vi "Get Maximum Button Width Vertical Toolbar.vi"(10 "Button Width":i32, 11 "All Icon Bounds":T1[](array[typedef])) -> (3 "Maximum Button Width":i32)   [LabVIEW 2011]
doc: "-------------\nDeveloped by Brian Hoover (hooovahh)"
uses:
  <vilib>/Utility/miscctls.llb/LVRectTypeDef.ctl
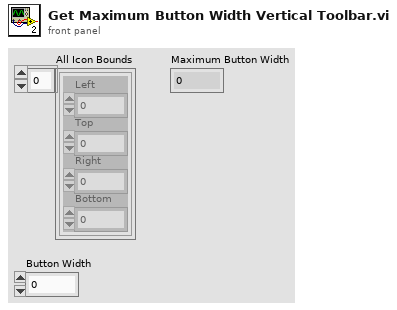
[diagram p1: front panel]
types:
  T1 = typedef "LVRectTypeDef.ctl" = cluster{"Left":i16, "Top":i16, "Right":i16, "Bottom":i16}
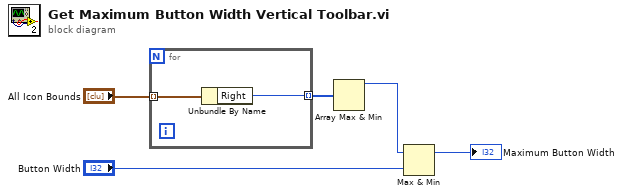
[diagram p0: block diagram]
diagram:
  n1 = for {
    tunnel: "All Icon Bounds" -> [w7] mode=indexing
    tunnel: [w6] -> w4 mode=indexing
    n2 = Unbundle By Name(w7) -> ("Right"=w6:i16)
  }
  n3 = Array Max & Min(array=w4) -> (max value=w3:i16)  [unwired: 3 out]
  n4 = Max & Min(x=w3, y="Button Width") -> (max(x,y)=→"Maximum Button Width":i32)  [unwired: 1 out]
